vi "Find Workspace.vi"(8 "error in (no error)":errorcluster, 10 "Control In":T2, 11 "Component.lvclass":refnum<class "Component Tray.lvclass">) -> (0 "error out":errorcluster, 1 "Workspace":T1, 2 "Control Out":T2, 3 "Workspace Out":refnum<class "Component Tray.lvclass">)   [LabVIEW 2019, in "Component Tray.lvclass"]
uses:
  Component Tray.lvclass
  Controller/Controllers.ctl
  Controller/I-O/I-O.lvclass
  Controller/Dispenser/Dispenser.lvclass
  C:/Program Files (x86)/Aerotech/A3200/LabVIEW/2010/Bin/Aerotech.A3200.dll
  Program Files (x86)/Aerotech/A3200/LabVIEW/2010/Bin/Aerotech.A3200.dll
  Workspace.ctl
  C:/Users/HEP/Documents/Aerotech gantry/UCSB-Gantry-master/V5/Classes/Workspace/Fixture.lvclass
  Fixture.lvclass/Fixture.ctl
  Read Fixture ID.vi
  Read Position.vi
  Fixture.lvclass
  Controller/Controller.lvclass
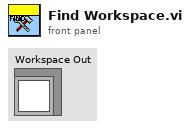
[diagram p1: front panel]
types:
  T1 = typedef "Fixture.lvclass/Workspace.ctl" = cluster{"XYZTheta":dbl[], "Workspace Valve":i32, "Workspace Sensor":i32}
  T2 = typedef "Controller.lvclass/Controllers.ctl" = cluster{"I-O.lvclass":refnum<class "I-O.lvclass">, "Dispenser.lvclass":refnum<class "Dispenser.lvclass">, "Gantry":refnum<k24>}
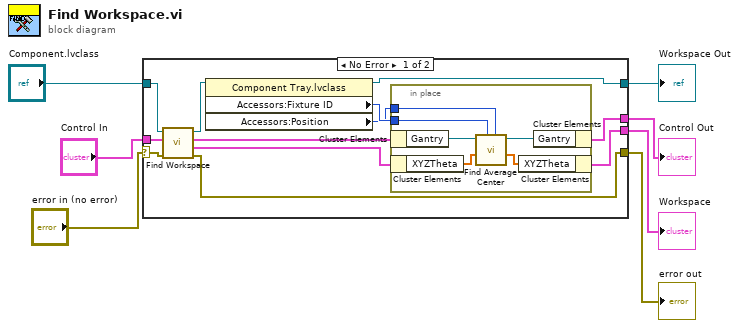
[diagram p0: block diagram]
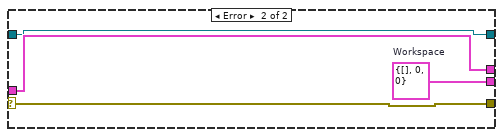
[diagram p2: hidden frame]
diagram:
  n1 = case shown="No Error" "error in (no error)" {
    selector: "error in (no error)" -> [w17 w29]
    tunnel: [w13 w28] -> w7
    tunnel: [w19 w29] -> w6
    tunnel: [w12 w27] -> w5
    tunnel: "Control In" -> [w16 w28]
    tunnel: [w8 w26] -> w2
    tunnel: "Component.lvclass" -> [w15 w26]
    frame No Error {
      n2 = call-parent "Find Workspace.vi"("Error In"=w17, "Control In"=w16, "Workspace In"=w15) -> ("Error Out"=w19:errorcluster, 1:"Workspace Out"=w18:T1, "Control Out"=w14:T2, 3:"Workspace Out"=w9:refnum<class "Component Tray.lvclass">)  [unwired: 5 in]
      n3 = property class="Component Tray.lvclass"(reference=w9) -> (reference out=w8:refnum<class "Component Tray.lvclass">, "Accessors:Fixture ID"=w11:i32, "Accessors:Position"=w10:i32)  [unwired: 1 in, 1 out]
      n4 = in-place {
        in-place-border: w11 -> [w23]
        in-place-border: w10 -> [w22]
        n5 = in-place-cluster #1(w14) -> ("Gantry"=w21:refnum<k24>)
        n6 = in-place-cluster #2(w18) -> ("XYZTheta"=w24:dbl[])
        n7 = call "Find Average Center.vi"("Position"=w22, "Tray Number"=w23, "XYZTheta"=w24, "Gantry In"=w21) -> ("XYZTheta"=w25:dbl[], "Gantry Out"=w20:refnum<k24>)  [unwired: 6 in]
        n8 = in-place-cluster #2("XYZTheta"=w25) -> (w12:T1)
        n9 = in-place-cluster #1("Gantry"=w20) -> (w13:T2)
      }
    }
    frame Error {
      w27 = T1 {"XYZTheta"=[], "Workspace Valve"=0, "Workspace Sensor"=0}  # Workspace
    }
  }
  "error out" <- w6
  "Control Out" <- w7
  "Workspace" <- w5
  "Workspace Out" <- w2
